vi "AUToscale.vi"(8 "Error":errorcluster caption="错误输入（无错误）", 10 "Delay Time (s)":dbl=1.0 caption="延迟时间(s)", 11 "VISA resource name":refnum<visa-resource-name>) -> (0 "Error out":errorcluster caption="错误输出", 3 "VISA resource name out":refnum<visa-resource-name>)   [LabVIEW 2020]
doc: "预设状态"
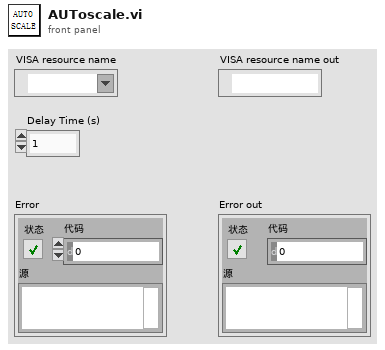
[diagram p1: front panel]
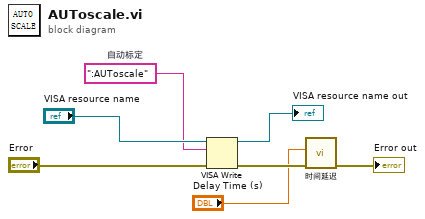
[diagram p0: block diagram]
diagram:
  w4 = ":AUToscale"  # 自动标定
  n1 = VISA Write(VISA resource name="VISA resource name", write buffer=w4, error in (no error)="Error") -> (VISA resource name out=→"VISA resource name out":refnum<visa-resource-name>, error out=w3:errorcluster)  [unwired: 1 out]
  n2 = call "时间延迟"("error in (no error)"=w3, "Delay Time (s)"="Delay Time (s)") -> ("error out"=→"Error out":errorcluster)  [unwired: 9 in]
